vi "Enable Data Acquisition.vi"(8 "error in (no error)":errorcluster, 10 "Enable Data Acquisition (Disable)":bool, 11 "VISA resource name":refnum<visa-resource-name>) -> (0 "error out":errorcluster, 3 "VISA resource name out":refnum<visa-resource-name>)   [LabVIEW 2020, in "Library Instrument & Equipement.lvlib" / "Library Multimeter.lvlib" / "RIGOL DM3058.lvlib"]
doc: "Enables or disables the data acquisition function.\n\n<B>Note:</B>\nThis VI only applies for RIGOL DM3051 model with firmware 03.12.00.03.04.00.07 or later."
uses:
  RIGOL DM3058.lvlib
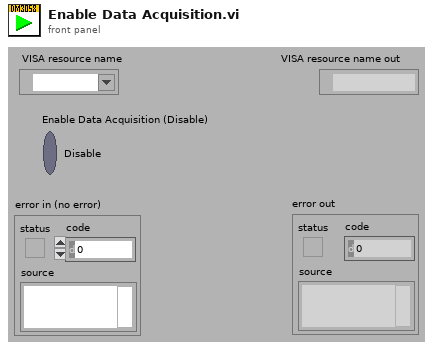
[diagram p1: front panel]
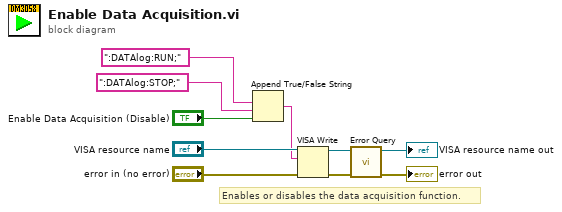
[diagram p0: block diagram]
diagram:
  # "Enables or disables the data acquisition function."
  n1 = Append True/False String(1:"Enable Data Acquisition (Disable)", 2:":DATAlog:STOP;" ("false string"), 3:":DATAlog:RUN;" ("true string")) -> (0:w8:string)  [unwired: 1 out]
  n2 = VISA Write(VISA resource name="VISA resource name", write buffer=w8, error in (no error)="error in (no error)") -> (VISA resource name out=w4:refnum<visa-resource-name>, error out=w3:errorcluster)  [unwired: 1 out]
  n3 = call "Error Query.vi"("error in (no error)"=w3, "VISA resource name"=w4) -> ("error out"=→"error out":errorcluster, "VISA resource name out"=→"VISA resource name out":refnum<visa-resource-name>)  [unwired: 6 in, 2 out]
